vi "Write.vi"(1 "error in (no error)":errorcluster, 2 "write buffer":string, 3 "VISA resource name":refnum<visa-resource-name>) -> (0 "error out":errorcluster)   [LabVIEW 2011]
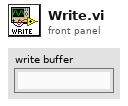
[diagram p1: front panel]
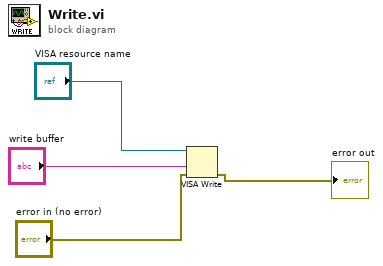
[diagram p0: block diagram]
diagram:
  n1 = VISA Write(VISA resource name="VISA resource name", write buffer="write buffer", error in (no error)="error in (no error)") -> (error out=→"error out":errorcluster)  [unwired: 2 out]
